vi "get target resources.vi"(8 "error in (no error)":errorcluster, 9 "get unmapped?":bool, 10 "get mapped?":bool, 11 "Item Ref in":T2 format="%.0x") -> (0 "error out":errorcluster, 3 "Array":T1[](array[typedef]) {"FPGA CD Ref" format="%.0x"; "reserver" format="%.0x"})   [LabVIEW 2016, in "RM.Server.lvlib"]
uses:
  RM.Server.lvlib
  <vilib>/NI Veristand/Custom Device API/Custom Device Item Ref.ctl
  viz_entry.ctl
  FPGA-Addon/Source/Shared/FG Action.ctl
  FPGA-Addon/Source/Shared/Constants.vi
  <vilib>/NI Veristand/Custom Device API/Get Item Property (Variant).vi
  <vilib>/NI Veristand/Custom Device API/NI VeriStand - Set Item Property.vi
  <vilib>/NI Veristand/Custom Device API/Set Item Property (Variant).vi
  <vilib>/NI Veristand/Custom Device API/Get Item Property (Dependent Node Pointer).vi
  <vilib>/NI Veristand/Custom Device API/Get Item Property (String).vi
  <vilib>/NI VeriStand/Custom Device API/Custom Device API.lvlib
  FPGA-Addon/Source/Shared/FPGA Addon Shared.lvlib
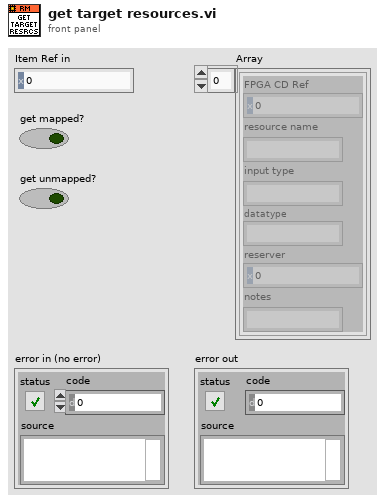
[diagram p1: front panel]
types:
  T1 = typedef "RM.Server.lvlib/viz_entry.ctl" = cluster{"FPGA CD Ref":T2, "resource name":string, "input type":string, "datatype":string, "reserver":T2, "notes":string}
  T2 = typedef "Custom Device API.lvlib/Custom Device Item Ref.ctl" = u64
  T3 = typedef "FPGA Addon Shared.lvlib/FG Action.ctl" = enum8{"GET", "SET"}
  T4 = typedef "Custom Device API.lvlib/Custom Device Item Info.ctl" = cluster{"Name":string, "Is Channel":bool, "GUID":string, "Is Waveform":bool}
  T5 = typedef "FPGA Addon Shared.lvlib/Register Information.ctl" = cluster{"Name":string, "Data Type":T6, "Default Value":variant}
  T6 = typedef "FPGA Addon Shared.lvlib/Data Type.ctl" = enum8{"<Null>", "I8", "I16", "I32", "I64", "U8", "U16", "U32", "U64", "SGL", "Boolean", "Analog PWM In Settings", "Analog PWM In", "Digital PWM In Settings", "Digital PWM In", "Digital PWM Out", "Sine Out", "FXP+/-24.5", "FXP+/-16.5", "FXP+/-32.8", "FXP+/-64.32", "FXP+/-16.7", "FXP+/-20.5"}
  T7 = typedef "Fifo_DMA_Config.ctl" = cluster{"Name":string, "Depth":u32, "Write? (Deprecated:Use Implementation)":bool, "Physical Channel":u32, "Base Address":u32, "Data Width":u32, "Data Type":T8, "FXP Properties":variant, "Write Window Address":u32, "Implementation":T9, "Control Set":u32}
  T8 = typedef "niFpgaDataTypeControl.ctl" = enum32{"Boolean", "I8", "I16", "I32", "I64", "U8", "U16", "U32", "U64", "FXP", "CustomControl", "SGL"}
  T9 = typedef "niFpgaDmaChannelImplementation.ctl" = enum16{"niFpgaTargetToHost", "niFpgaHostToTarget", "niFpgaPeerToPeerWriter", "niFpgaPeerToPeerReader", "niCoreTargetToHost", "niCoreHostToTarget"}
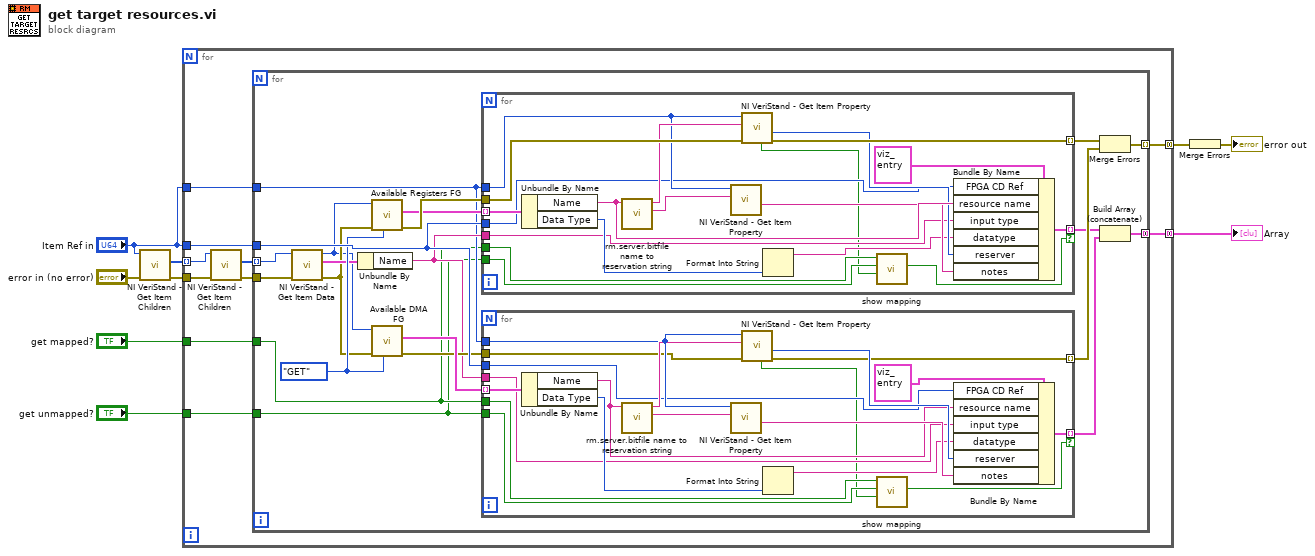
[diagram p0: block diagram]
diagram:
  n1 = call <vilib>:"NI VeriStand - Get Item Children.vi"("error in (no error)"="error in (no error)", "Item Ref in"="Item Ref in") -> ("error out"=w3:errorcluster, "Child Refs"=w4:T2[])  [unwired: 6 in, 2 out]
  n2 = for {
    tunnel: w3 -> [w18]
    tunnel: w4 -> [w16] mode=indexing
    tunnel: "Item Ref in" -> [w15]
    tunnel: [w14] -> w5 mode=concatenating
    tunnel: [w13] -> w6 mode=concatenating
    tunnel: "Item Ref in" -> [w12]
    tunnel: "get mapped?" -> [w11]
    tunnel: "get unmapped?" -> [w10]
    n3 = call <vilib>:"NI VeriStand - Get Item Children.vi"("error in (no error)"=w18, "Item Ref in"=w16) -> ("error out"=w17:errorcluster, "Child Refs"=w19:T2[])  [unwired: 6 in, 2 out]
    n4 = for {
      tunnel: w17 -> [w26]
      tunnel: w19 -> [w29] mode=indexing
      tunnel: w15 -> [w22]
      tunnel: [w34] -> w14 mode=indexing
      tunnel: [w31] -> w13 mode=concatenating
      tunnel: w12 -> [w37]
      tunnel: w11 -> [w21]
      tunnel: w10 -> [w20]
      w30 = FG_Action."GET" ("Action")
      n5 = call <vilib>:"NI VeriStand - Get Item Data.vi"("error in (no error)"=w26, "Item Ref in"=w29) -> ("error out"=w25:errorcluster, "Item Info"=w28:T4, "Item Ref out"=w23:T2)  [unwired: 6 in, 1 out]
      n6 = Unbundle By Name(w28) -> ("Name"=w24:string)
      n7 = call "Available Registers FG.vi"("Action"=w30, "error in (no error)"=w25, "Item Ref"=w23) -> ("error out"=w40:errorcluster, "Available Registers"=w39:T5[])  [unwired: 6 in, 1 out]
      n8 = call "Available DMA FG.vi"("Action"=w30, "error in (no error)"=w25, "Item Ref"=w23) -> ("error out"=w27:errorcluster, "Available DMA"=w38:T7[])  [unwired: 6 in, 1 out]
      n9 = for {
        tunnel: w39 -> [w78] mode=indexing
        tunnel: w22 -> [w75]
        tunnel: w40 -> [w77]
        tunnel: [w73] -> w36 mode=indexing
        tunnel: [w67] -> w33 mode=indexing if=w60
        tunnel: w37 -> [w66]
        tunnel: w24 -> [w64]
        tunnel: w21 -> [w63]
        tunnel: w20 -> [w62]
        n10 = Unbundle By Name(w78) -> ("Name"=w71:string, "Data Type"=w70:T6)
        n11 = call "rm.server.bitfile name to reservation string.vi"("Name in bitfile"=w71) -> ("Notes String"=w74:string, "Reservation String"=w76:string)  [unwired: 9 in]
        n12 = call-poly <vilib>:"NI VeriStand - Get Item Property.vi"("Property Name"=w74, "Item Ref in"=w75) -> ("Value"=w68:string)  [unwired: 6 in, 3 out]
        n13 = call-poly <vilib>:"NI VeriStand - Get Item Property.vi"("error in (no error)"=w77, "Property Name"=w76, "Item Ref in"=w75) -> ("error out"=w73:errorcluster, "Dependent Node Ref"=w69:T2, "Found"=w61:bool)  [unwired: 5 in, 1 out]
        n14 = Format Into String(w70) -> (resulting string=w65:string)  [unwired: 3 in, 1 out]
        n15 = call "show mapping"("is mapped?"=w61, "show unmapped?"=w62, "show mapped?"=w63) -> ("show?"=w60:bool)  [unwired: 8 in]
        n16 = Bundle By Name(cluster=T1 {"FPGA CD Ref"=18446744073709551615, "resource name"="", "input type"="", "datatype"="", "reserver"=18446744073709551615, "notes"=""} ("visualizer entry"), "FPGA CD Ref"=w66, "resource name"=w71, "input type"=w64, "datatype"=w65, "reserver"=w69, "notes"=w68) -> (w67:T1)
      }
      n17 = for {
        tunnel: w38 -> [w54] mode=indexing
        tunnel: w22 -> [w53]
        tunnel: w37 -> [w52]
        tunnel: w27 -> [w51]
        tunnel: [w50] -> w35 mode=indexing
        tunnel: [w47] -> w32 mode=indexing if=w41
        tunnel: w24 -> [w46]
        tunnel: w21 -> [w44]
        tunnel: w20 -> [w43]
        n18 = Unbundle By Name(w54) -> ("Name"=w45:string, "Data Type"=w49:T8)
        n19 = call "rm.server.bitfile name to reservation string.vi"("Name in bitfile"=w45) -> ("Notes String"=w56:string, "Reservation String"=w55:string)  [unwired: 9 in]
        n20 = call-poly <vilib>:"NI VeriStand - Get Item Property.vi"("Property Name"=w56, "Item Ref in"=w53) -> ("Value"=w59:string)  [unwired: 6 in, 3 out]
        n21 = call-poly <vilib>:"NI VeriStand - Get Item Property.vi"("error in (no error)"=w51, "Property Name"=w55, "Item Ref in"=w53) -> ("error out"=w50:errorcluster, "Dependent Node Ref"=w58:T2, "Found"=w42:bool)  [unwired: 5 in, 1 out]
        n22 = Format Into String(w49) -> (resulting string=w48:string)  [unwired: 3 in, 1 out]
        n23 = call "show mapping"("is mapped?"=w42, "show unmapped?"=w43, "show mapped?"=w44) -> ("show?"=w41:bool)  [unwired: 8 in]
        n24 = Bundle By Name(cluster=T1 {"FPGA CD Ref"=18446744073709551615, "resource name"="", "input type"="", "datatype"="", "reserver"=18446744073709551615, "notes"=""} ("visualizer entry"), "FPGA CD Ref"=w52, "resource name"=w45, "input type"=w46, "datatype"=w48, "reserver"=w58, "notes"=w59) -> (w47:T1)
      }
      n25 = Merge Errors(w36, w35) -> (w34:errorcluster)
      n26 = Build Array (concatenate)(w33, w32) -> (w31:T1[])
    }
  }
  "Array" <- w6
  n27 = Merge Errors(w5) -> (→"error out":errorcluster)
